vi "Fix Angle.vi"(11 "Angle In":dbl) -> (3 "Angle Out":dbl)   [LabVIEW 2016]
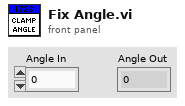
[diagram p1: front panel]
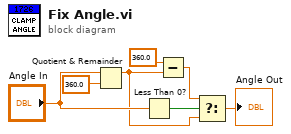
[diagram p0: block diagram]
diagram:
  n1 = Quotient & Remainder(x="Angle In", y=360.0) -> (x-y*floor(x/y)=w2:dbl)  [unwired: 1 out]
  n2 = Less Than 0?(x="Angle In") -> (x < 0?=w1:bool)
  n3 = Subtract(x=360.0 ("y"), y=w2) -> (x-y=w3:dbl)
  n4 = Select(t=w3, s=w1, f=w2) -> (s? t:f=→"Angle Out":dbl)
